vi "stack_dropn.vi"(8 "error in (no error)":errorcluster, 10 "n":i32=1, 11 "Lua in":refnum<class "Lua.lvclass">) -> (0 "error out":errorcluster, 3 "Lua out":refnum<class "Lua.lvclass">)   [LabVIEW 2020, in "Lua for LabVIEW.lvlib" / "Lua.lvclass"]
doc: "Drops N items from the stack. (equivalent to lua_settop(-(N+1))"
uses:
  Lua.lvclass
  Lua.lvclass/Lua.ctl
  lib/lua.dll/lua.dll.lvlib
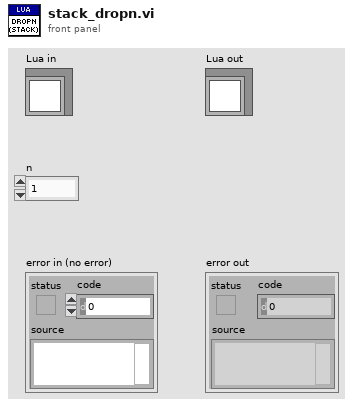
[diagram p1: front panel]
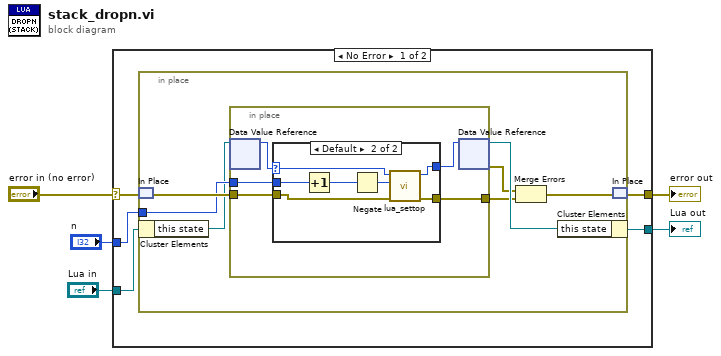
[diagram p0: block diagram]
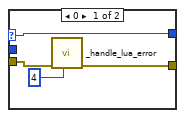
[diagram p2: hidden frame]
diagram:
  n1 = case shown="No Error" "error in (no error)" {
    selector: "error in (no error)" -> [w7 w35]
    tunnel: [w8 w35] -> w4
    tunnel: [w9 w34] -> w2
    tunnel: "Lua in" -> [w10 w34]
    tunnel: "n" -> [w6 _]
    frame No Error {
      n2 = in-place {
        in-place-border: w6 -> [w16]
        n3 = in-place-match #1(w7) -> (w17:errorcluster)
        n4 = in-place-cluster #2(w10) -> ("this state"=w15:refnum<data-value>)
        n5 = in-place {
          in-place-border: w17 -> [w22]
          in-place-border: [w21] -> w12
          in-place-border: w16 -> [w20]
          n6 = in-place-dvr #3(w15) -> (w19:u64)  [unwired: 1 out]
          n7 = case shown="Default" w19 {
            selector: w19 -> [w26 w33]
            tunnel: [w26 w32] -> w18
            tunnel: w22 -> [w23 w30]
            tunnel: [w24 w31] -> w21
            tunnel: w20 -> [_ w28]
            frame 0 {
              n8 = call "_handle_lua_error.vi"("lua status"=4 ("lua_load errcode"), "error in (no error)"=w23) -> ("error out"=w24:errorcluster)  [unwired: 9 in]
            }
            frame Default {
              n9 = Increment(x=w28) -> (x+1=w27:i32)
              n10 = Negate(x=w27) -> (-x=w29:i32)
              n11 = call "lua_settop.vi"("error in (no error)"=w30, "index"=w29, "lua_state_p"=w33) -> ("error out"=w31:errorcluster, "lua_state_p out"=w32:u64)  [unwired: 7 in]
            }
          }
          n12 = in-place-dvr #3(w18) -> (w14:refnum<data-value>, w13:errorcluster)
        }
        n13 = Merge Errors(w13, w12) -> (w11:errorcluster)
        n14 = in-place-cluster #2("this state"=w14) -> (w9:refnum<class "Lua.lvclass">)
        n15 = in-place-match #1(w11) -> (w8:errorcluster)
      }
    }
    frame Error {
    }
  }
  "error out" <- w4
  "Lua out" <- w2
